vi "build local designator settings string (MAK).vi"(10 "configuration string":string, 11 "configuration file":path) -> (3 "local designator settings":string)   [LabVIEW 2019, in "HLA Custom Device Engine.lvlib"]
uses:
  HLA Custom Device Engine.lvlib
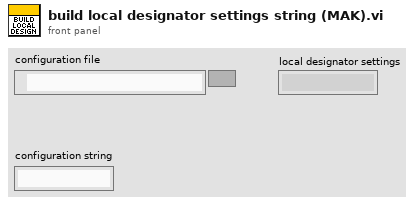
[diagram p1: front panel]
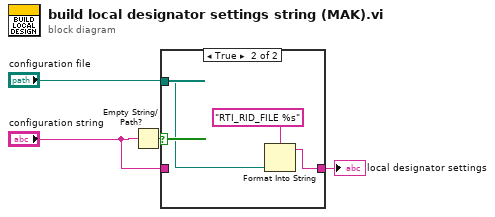
[diagram p0: block diagram]
diagram:
  n1 = Empty String/Path?(string/path="configuration string") -> (empty?=w4:bool)
  n2 = case shown="True" w4 {
    tunnel: "configuration string" -> [w5 _]
    tunnel: [w5 w7] -> w2
    tunnel: "configuration file" -> [_ w6]
    frame False {
    }
    frame True {
      n3 = Format Into String(format string="RTI_RID_FILE %s", w6) -> (resulting string=w7:string)  [unwired: 2 in, 1 out]
    }
  }
  "local designator settings" <- w2
